vi "Read Message.vi"(6 "timeout in ms (100)":i32=100, 8 "error in (no error)":errorcluster, 10 "index":i32, 11 "RemoteControl.ZMQ in":refnum<class "RemoteControl.ZMQ.lvclass">) -> (0 "error out":errorcluster, 1 "Data":variant, 2 "Command":string, 3 "RemoteControl.ZMQ out":refnum<class "RemoteControl.ZMQ.lvclass">, 4 "ID":string)   [LabVIEW 2019, in "RemoteControl.ZMQ.lvclass"]
uses:
  RemoteControl.ZMQ.lvclass
  C:/Users/patrick/Documents/GitHub/Instrument-Framework/lvsrc/SMOs/RemoteControl/RemoteControl.lvclass
  RemoteControl.ZMQ.lvclass/RemoteControl.ZMQ.ctl
  RemoteControl/Typedefs/Message--Cluster.ctl
  RemoteControl/RemoteControl.lvclass/RemoteControl.ctl
  <vilib>/Utility/error.llb/Error Cluster From Error Code.vi
  <vilib>/ErrorRing/Error Ring.xnode
  RemoteControl/RemoteControl.lvclass
  <vilib>/addons/zeromq/zmq_socket.lvclass
  JSON-RPC/JSON-RPC/JSON-RPC.lvclass
  <vilib>/addons/zeromq/zmq_context.lvclass
panel:
  out "Numeric":i32
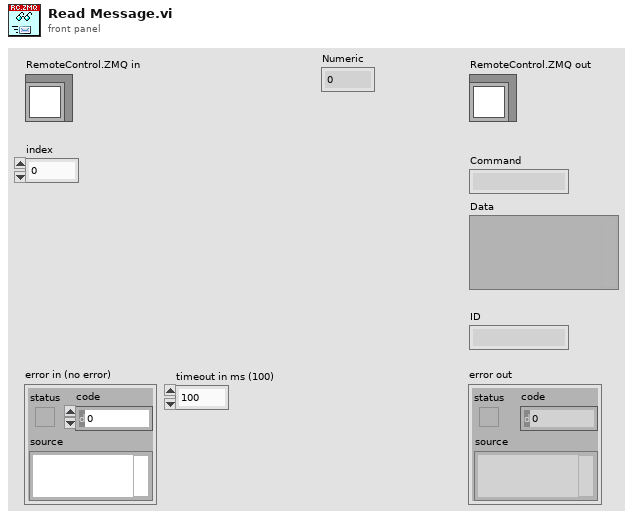
[diagram p1: front panel]
types:
  T1 = typedef "RemoteControl.lvclass/Message--Cluster.ctl" = cluster{"Command":string, "Data":variant, "ID":string}
  T2 = typedef "zeromq.lvlib/socket_type.ctl" = enum8{"ZMQ_PAIR", "ZMQ_PUB", "ZMQ_SUB", "ZMQ_REQ", "ZMQ_REP", "ZMQ_DEALER", "ZMQ_ROUTER", "ZMQ_PULL", "ZMQ_PUSH", "ZMQ_XPUB", "ZMQ_XSUB"}
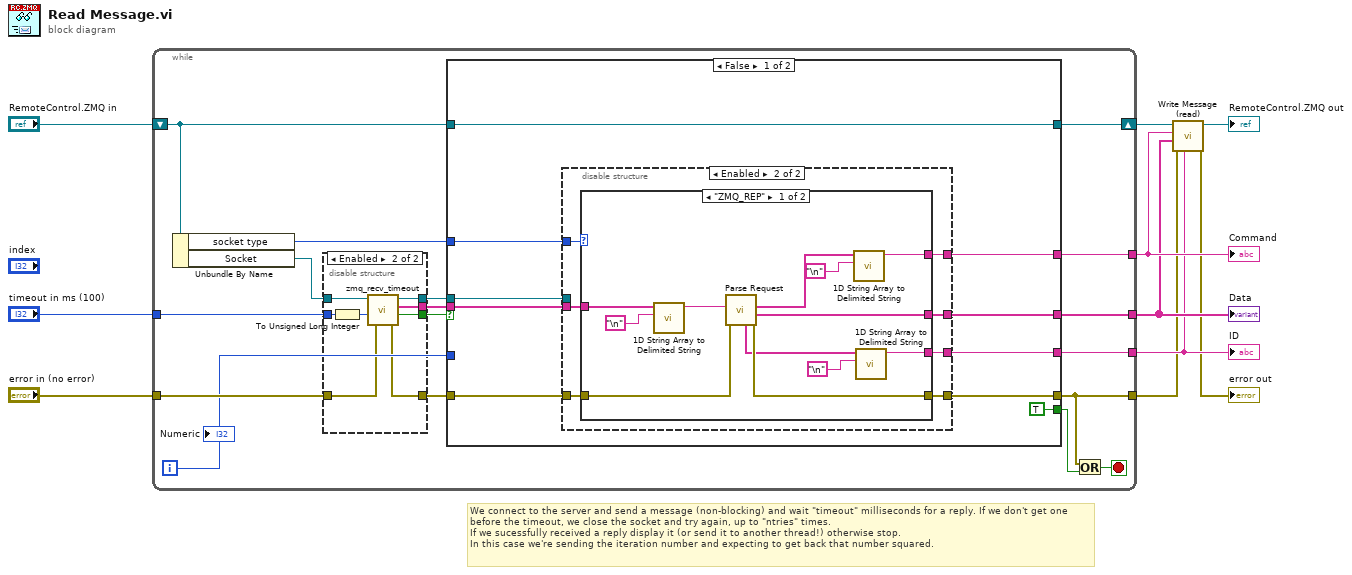
[diagram p0: block diagram]
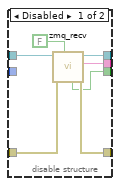
[diagram p2: hidden frame]
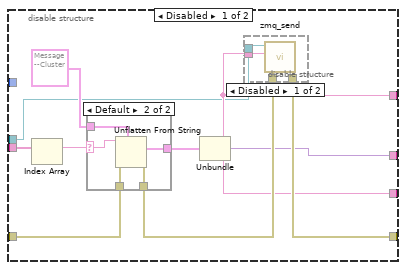
[diagram p3: hidden frame]
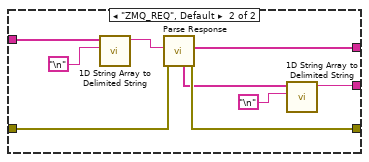
[diagram p6: hidden frame]
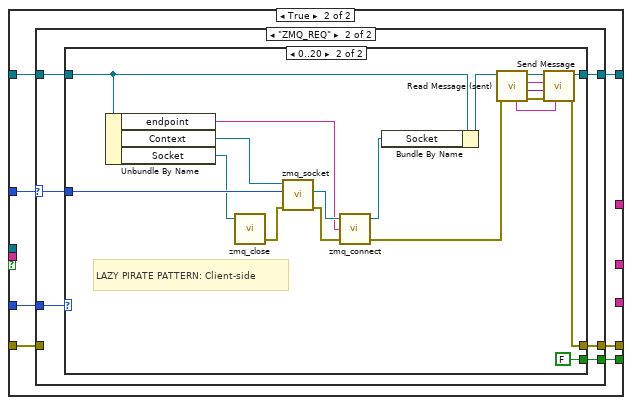
[diagram p7: hidden frame]
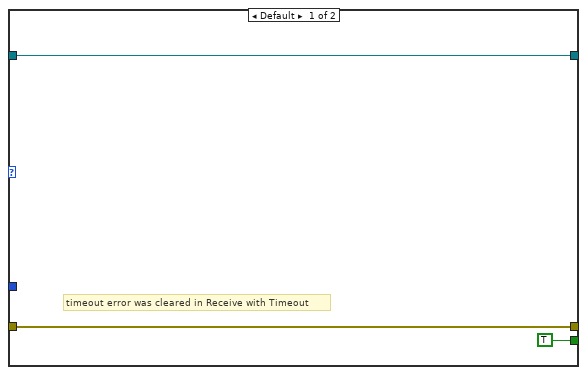
[diagram p8: hidden frame]
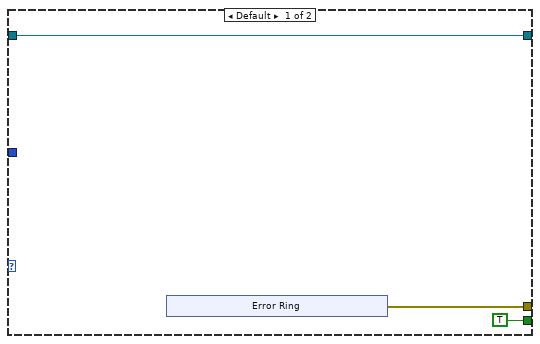
[diagram p9: hidden frame]
diagram:
  # "We connect to the server and send a message (non-blocking) and wait \"timeout\" milliseconds for a reply. If we don't get one before the timeout, we close the socket and try again, up to \"ntries\" times.\nIf we sucessfully received a reply display it (or send it to another thread!) otherwise stop.\nIn this case we're sending the iteration number and expecting to get back that number squared."
  n1 = while {
    tunnel: [w23] -> w8
    tunnel: [w22] -> w7
    tunnel: [w21] -> w6
    tunnel: "timeout in ms (100)" -> [w19]
    tunnel: "error in (no error)" -> [w27]
    tunnel: [w12] -> w5
    shift-right: [w15] -> w1
    shift-left: "RemoteControl.ZMQ in" -> [w18]
    i -> [w14]
    stop <- w13 stop-if-true
    n2 = Unbundle By Name(w18) -> ("socket type"=w17:T2, "Socket"=w16:refnum<class "zmq_socket.lvclass">)
    n3 = disable-structure shown="Enabled" {
      disable-tunnel: w27 -> [w34 w38]
      disable-tunnel: [w33 w37] -> w26
      disable-tunnel: [w32 w41] -> w25
      disable-tunnel: [w31 w40] -> w24
      disable-tunnel: w16 -> [w30 w39]
      disable-tunnel: [w28 w42] -> w20
      disable-tunnel: w19 -> [_ w36]
      frame Disabled {
        n4 = call <vilib>:"zmq_recv.vi"("no block? (F)"=FALSE, "error in"=w34, "socket in"=w30) -> ("error out"=w33:errorcluster, "data"=w31:string, "socket out"=w32:refnum<class "zmq_socket.lvclass">, "timeout?"=w28:bool)  [unwired: 2 in, 1 out]
      }
      frame Enabled {
        n5 = To Unsigned Long Integer(number=w36) -> (unsigned 32bit integer=w35:u32)
        n6 = call <vilib>:"zmq_recv_timeout.vi"("error in"=w38, "timeout (ms)"=w35, "socket in"=w39) -> ("error out"=w37:errorcluster, "timeout?"=w42:bool, "parts"=w40:string[], "socket out"=w41:refnum<class "zmq_socket.lvclass">)  [unwired: 1 in]
      }
    }
    n7 = case shown="False" w20 {
      tunnel: [w52 _] -> w22
      tunnel: [w51 _] -> w21
      tunnel: [w50 _] -> w23
      tunnel: w26 -> [w49 w108]
      tunnel: w25 -> [w48 _]
      tunnel: w24 -> [w47 _]
      tunnel: w17 -> [w46 w109]
      tunnel: w18 -> [w45 w110]
      tunnel: [w45 w107] -> w15
      tunnel: w14 -> [_ w106]
      tunnel: [w44 w105] -> w12
      tunnel: [TRUE w104] -> w11
      frame False {
        n8 = disable-structure shown="Enabled" {
          disable-tunnel: [w63 w79] -> w44
          disable-tunnel: [w56 w77] -> w52
          disable-tunnel: [w55 w76] -> w51
          disable-tunnel: [w62 w78] -> w50
          disable-tunnel: w49 -> [w60 w80]
          disable-tunnel: w48 -> [w53 _]
          disable-tunnel: w47 -> [w58 w81]
          disable-tunnel: w46 -> [_ w82]
          frame Disabled {
            n9 = Index Array(array=w58) -> (element=w54:string)  [unwired: 1 in]
            n10 = case shown="Default" w54 {
              selector: w54 -> [_ w71]
              tunnel: T1 {"Command"="", "Data"=variant, "ID"=""} ("Message") -> [w69 w72]
              tunnel: [w69 w75] -> w61
              tunnel: w60 -> [w70 w74]
              tunnel: [w70 w73] -> w59
              frame "" {
              }
              frame Default {
                n11 = Unflatten From String(type=w72, binary string=w71, error in (no error)=w74) -> (value=w75:T1, error out=w73:errorcluster)  [unwired: 2 in, 1 out]
              }
            }
            n12 = Unbundle(w61) -> ("Command"=w62:string, "Data"=w56:variant, "ID"=w55:string)
            n13 = disable-structure shown="Disabled" {
              disable-tunnel: [w67 w68] -> w63
              disable-tunnel: w62 -> [w66 _]
              disable-tunnel: w59 -> [w65 w68]
              disable-tunnel: w53 -> [w64 _]
              frame Disabled {
                n14 = call <vilib>:"zmq_send.vi"("error in"=w65, "data"=w66, "socket in"=w64) -> ("error out"=w67:errorcluster)  [unwired: 4 in, 1 out]
              }
              frame Enabled {
              }
            }
          }
          frame Enabled {
            n15 = case shown="\"ZMQ_REP\"" w82 {
              tunnel: w81 -> [w83 w95]
              tunnel: w80 -> [w94 w103]
              tunnel: [w93 w102] -> w79
              tunnel: [w90 _] -> w78
              tunnel: [w92 w101] -> w77
              tunnel: [w86 w98] -> w76
              frame "ZMQ_REP" {
                n16 = call <vilib>:"1D String Array to Delimited String.vi"("delimiter"="\n", "string array"=w83) -> ("delimited string"=w84:string)  [unwired: 9 in]
                n17 = call "Parse Request.vi"("error in (no error)"=w94, "{JSON} Request"=w84) -> ("error out"=w93:errorcluster, "Params"=w92:string[], "Methods"=w91:string[], "IDs"=w87:string[])  [unwired: 5 in, 1 out]
                n18 = call <vilib>:"1D String Array to Delimited String.vi"("delimiter"="\n", "string array"=w91) -> ("delimited string"=w90:string)  [unwired: 9 in]
                n19 = call <vilib>:"1D String Array to Delimited String.vi"("delimiter"="\n", "string array"=w87) -> ("delimited string"=w86:string)  [unwired: 9 in]
              }
              frame "ZMQ_REQ", Default {
                n20 = call <vilib>:"1D String Array to Delimited String.vi"("delimiter"="\n", "string array"=w95) -> ("delimited string"=w97:string)  [unwired: 9 in]
                n21 = call "Parse Response.vi"("error in (no error)"=w103, "{JSON} Response"=w97) -> ("error out"=w102:errorcluster, "results"=w101:string[], "IDs"=w100:string[])  [unwired: 5 in, 2 out]
                n22 = call <vilib>:"1D String Array to Delimited String.vi"("delimiter"="\n", "string array"=w100) -> ("delimited string"=w98:string)  [unwired: 9 in]
              }
            }
          }
        }
      }
      frame True {
        n23 = case shown="\"ZMQ_REQ\"" w109 {
          selector: w109 -> [_ w118]
          tunnel: w110 -> [w113 w119]
          tunnel: w108 -> [w112 _]
          tunnel: [w113 w117] -> w107
          tunnel: w106 -> [_ w114]
          tunnel: [w112 w116] -> w105
          tunnel: [TRUE w115] -> w104
          frame Default {
            # "timeout error was cleared in Receive with Timeout"
          }
          frame "ZMQ_REQ" {
            n24 = case shown="0..20" w114 {
              tunnel: w119 -> [w122 w141]
              tunnel: w118 -> [_ w140]
              tunnel: [w122 w134] -> w117
              tunnel: [w121 w128] -> w116
              tunnel: [TRUE FALSE] -> w115
              frame Default {
                n25 = xnode "Error Ring"() -> ("error out"=w121:errorcluster)
              }
              frame 0..20 {
                # "LAZY PIRATE PATTERN: Client-side"
                n26 = Unbundle By Name(w141) -> ("endpoint"=w138:string, "Context"=w142:refnum<class "zmq_context.lvclass">, "Socket"=w139:refnum<class "zmq_socket.lvclass">)
                n27 = call <vilib>:"zmq_close.vi"("socket"=w139) -> ("error out"=w145:errorcluster)  [unwired: 4 in]
                n28 = call <vilib>:"zmq_socket.vi"("error in"=w145, "socket type"=w140, "context in"=w142) -> ("error out"=w144:errorcluster, "socket out"=w143:refnum<class "zmq_socket.lvclass">)  [unwired: 2 in, 1 out]
                n29 = call <vilib>:"zmq_connect.vi"("error in"=w144, "endpoint"=w138, "socket in"=w143) -> ("error out"=w130:errorcluster, "socket out"=w137:refnum<class "zmq_socket.lvclass">)  [unwired: 1 in]
                n30 = Bundle By Name(cluster=w141, "Socket"=w137) -> (w136:refnum<class "RemoteControl.ZMQ.lvclass">)
                n31 = call "Read Message (sent).vi"("error in (no error)"=w130, "RemoteControl in"=w136) -> ("error out"=w131:errorcluster, "Data (Sent)"=w132:variant, "Command (Sent)"=w133:string, "RemoteControl out"=w135:refnum<class "RemoteControl.ZMQ.lvclass">, "ID (Sent)"=w129:string)  [unwired: 5 in]
                n32 = call-dynamic "Send Message.vi"("ID"=w129, "error in (no error)"=w131, "Data"=w132, "Command"=w133, "RemoteControl.ZMQ in"=w135) -> ("error out"=w128:errorcluster, "RemoteControl.ZMQ out"=w134:refnum<class "RemoteControl.ZMQ.lvclass">)  [unwired: 4 in, 1 out]
              }
            }
          }
        }
      }
    }
    n33 = Or(x=w12, y=w11) -> (x .or. y?=w13:bool)
    "Numeric" <- w14
  }
  "ID" <- w6
  "Command" <- w8
  "Data" <- w7
  n34 = call "Write Message (read).vi"("ID (Read)"=w6, "error in (no error)"=w5, "Data (Read)"=w7, "Command (Read)"=w8, "RemoteControl in"=w1) -> ("error out"=→"error out":errorcluster, "RemoteControl out"=→"RemoteControl.ZMQ out":refnum<class "RemoteControl.ZMQ.lvclass">)  [unwired: 5 in]
